vi "Write Channel names.vi"(8 "error in (no error)":errorcluster, 10 "Channel names":string[](array[string]), 11 "Find Peaks Result in":refnum<class "Find Peaks Result.lvclass">) -> (0 "error out":errorcluster, 3 "Find Peaks Result out":refnum<class "Find Peaks Result.lvclass">)   [LabVIEW 2015, in "Find Peaks Result.lvclass"]
uses:
  Find Peaks Result.lvclass
  Find Peaks Result.lvclass/Find Peaks Result.ctl
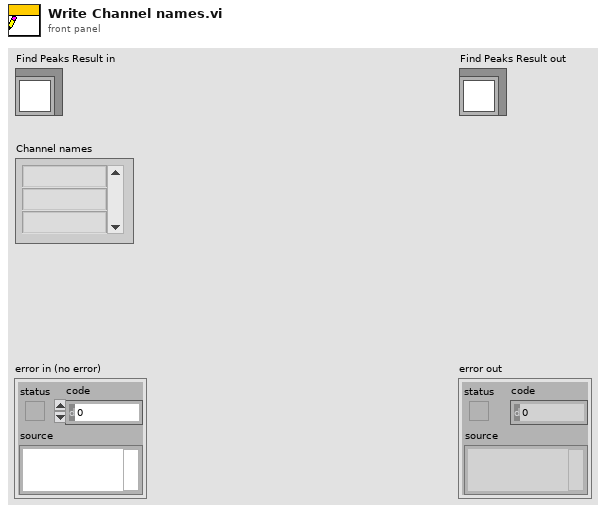
[diagram p1: front panel]
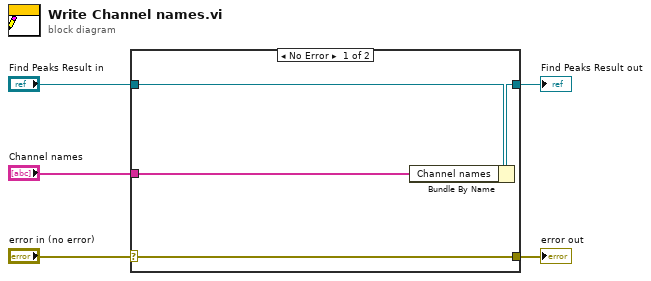
[diagram p0: block diagram]
diagram:
  n1 = case shown="No Error" "error in (no error)" {
    selector: "error in (no error)" -> [w9 w10]
    tunnel: [w9 w10] -> w4
    tunnel: [w7 w11] -> w2
    tunnel: "Find Peaks Result in" -> [w8 w11]
    tunnel: "Channel names" -> [w6 _]
    frame No Error {
      n2 = Bundle By Name(cluster=w8, "Channel names"=w6) -> (w7:refnum<class "Find Peaks Result.lvclass">)
    }
    frame Error {
    }
  }
  "error out" <- w4
  "Find Peaks Result out" <- w2
